vi "Set window name.vi"(8 "error in (no error)":errorcluster, 11 "LV MDI in":refnum<class "LV MDI.lvclass">) -> (0 "error out":errorcluster, 3 "LV MDI out":refnum<class "LV MDI.lvclass">)   [LabVIEW 2016, in "LV MDI.lvclass"]
uses:
  LV MDI.lvclass
  LV MDI.lvclass/LV MDI.ctl
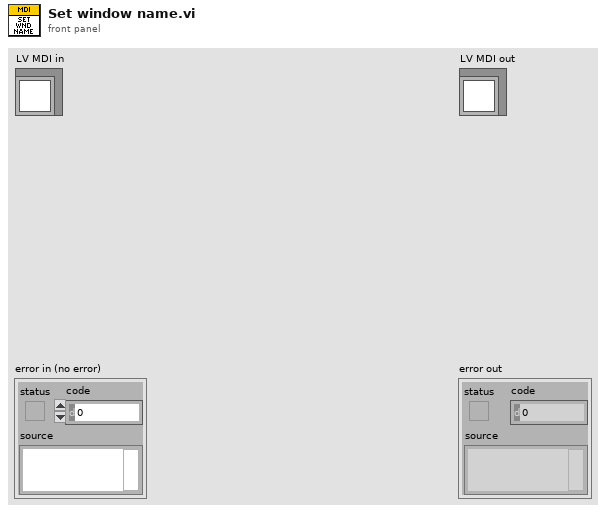
[diagram p1: front panel]
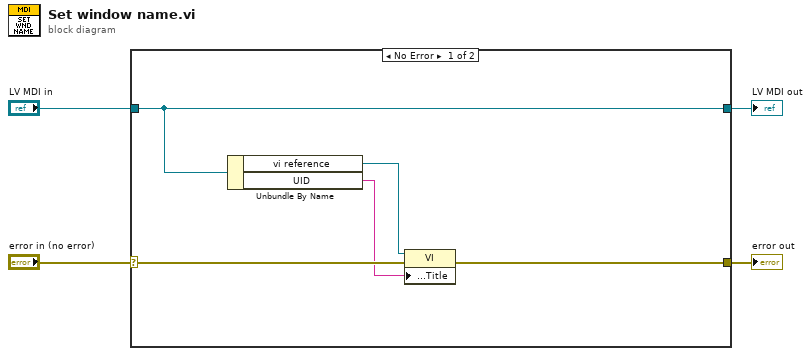
[diagram p0: block diagram]
diagram:
  n1 = case shown="No Error" "error in (no error)" {
    selector: "error in (no error)" -> [w9 w11]
    tunnel: [w7 w11] -> w3
    tunnel: [w8 w10] -> w1
    tunnel: "LV MDI in" -> [w8 w10]
    frame No Error {
      n2 = Unbundle By Name(w8) -> ("vi reference"=w5:refnum<vi>, "UID"=w6:string)
      n3 = property class="VI"(reference=w5, error in=w9, "Front Panel.Title"=w6) -> (error out=w7:errorcluster)  [unwired: 1 out]
    }
    frame Error {
    }
  }
  "error out" <- w3
  "LV MDI out" <- w1
